vi "XNET String To IO Name (Database Filepath).vi"(3 "filepath":path) -> (0 "XNET Database":refnum<k21>)   [LabVIEW 2018]
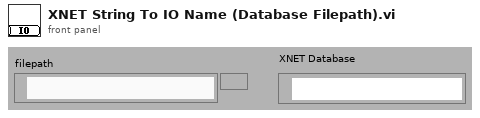
[diagram p1: front panel]
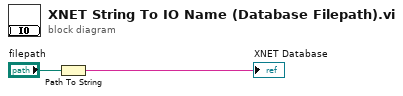
[diagram p0: block diagram]
diagram:
  n1 = Path To String(path="filepath") -> (string=→"XNET Database":string)
